vi "Utility_getSettings.vi"(8 "error in":errorcluster, 10 "Search Setting String":string) -> (0 "errorout":errorcluster, 2 "Setting Value":string, 3 "Found setting":bool)   [LabVIEW 2009, in "Utility.lvlib"]
uses:
  Utility.lvlib
panel:
  out "Array":string[](array[string])
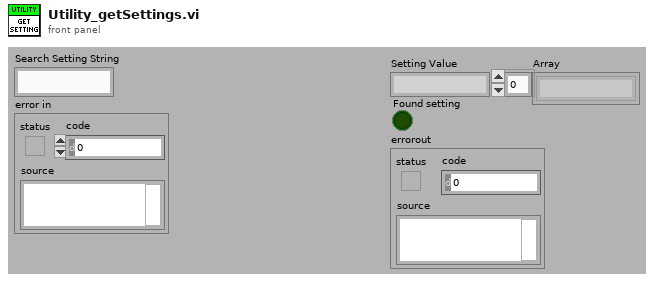
[diagram p1: front panel]
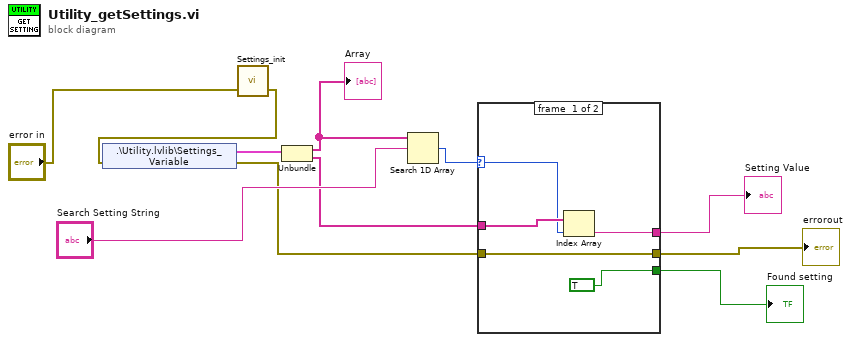
[diagram p0: block diagram]
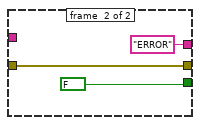
[diagram p2: hidden frame]
diagram:
  n1 = call "Settings_init.vi"("error in"="error in") -> ("error out"=w1:errorcluster)  [unwired: 2 in]
  n2 = shared-variable ".\\Utility.lvlib\\Settings_Variable"(error in=w1) -> (w11:cluster{string[], string[]}, error out=w8:errorcluster)
  n3 = Unbundle(w11) -> (w6:string[], w7:string[])
  "Array" <- w6
  n4 = Search 1D Array(1D array=w6, element="Search Setting String") -> (index of element=w9:i32)  [unwired: 1 in]
  n5 = case shown="0, Default" w9 {
    selector: w9 -> [w15 _]
    tunnel: w8 -> [w12 w17]
    tunnel: w7 -> [w16 _]
    tunnel: [w14 "ERROR" ("value")] -> w5
    tunnel: [TRUE FALSE] -> w4
    tunnel: [w12 w17] -> w3
    frame #0 {
      n6 = Index Array(array=w16, index=w15) -> (element=w14:string)
    }
    frame #1 {
    }
  }
  "Setting Value" <- w5
  "Found setting" <- w4
  "errorout" <- w3
